vi "ROV_IO 2 (SubVI).vi"(11 "ROV string":string="34.5,,,,$56.3,34.556,,,,$67.9") -> (3 "ROV OK":string)   [LabVIEW 2014]
panel:
  out "ROV temp":string
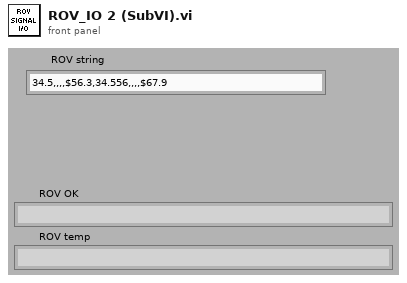
[diagram p1: front panel]
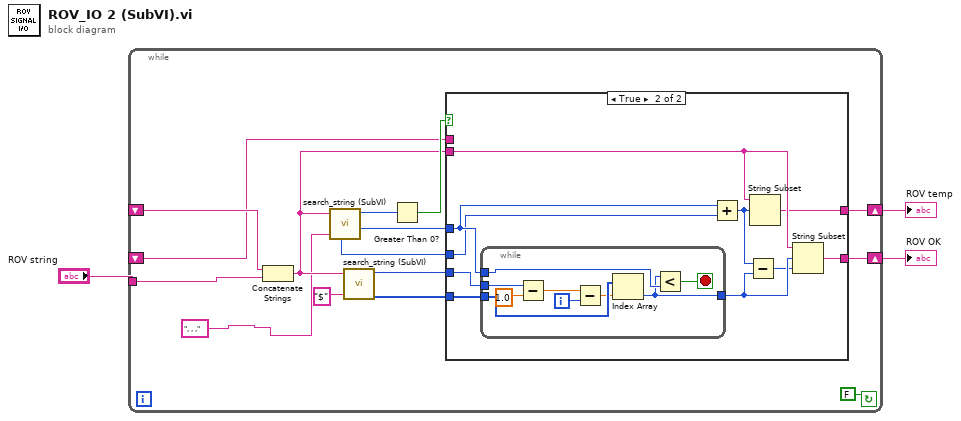
[diagram p0: block diagram]
diagram:
  n1 = while {
    tunnel: "ROV string" -> [w5]
    shift-right: [w9] -> w2
    shift-left: _ -> [w6]
    shift-right: [w8] -> w1
    shift-left: _ -> [w7]
    stop <- FALSE continue-if-true
    n2 = Concatenate Strings(w7, w5) -> (w11:string)
    n3 = call "search_string (SubVI).vi"("string"=w11, "search string/char (-)"=", , ,") -> ("search length"=w10:i32, "no. hits"=w16:i32, "pos last"=w12:i32)  [unwired: 6 out]
    n4 = call "search_string (SubVI).vi"("string"=w11, "search string/char (-)"="$") -> ("no. hits"=w14:i32, "pos vec"=w13:i32[])  [unwired: 7 out]
    n5 = Greater Than 0?(x=w16) -> (x > 0?=w15:bool)
    n6 = case shown="True" w15 {
      tunnel: w14 -> [_ w29]
      tunnel: w13 -> [_ w30]
      tunnel: w12 -> [_ w28]
      tunnel: w11 -> [w19 w23]
      tunnel: w10 -> [_ w27]
      tunnel: [w20 w24] -> w9
      tunnel: [w19 w22] -> w8
      tunnel: w6 -> [w20 _]
      frame False {
      }
      frame True {
        n7 = while {
          tunnel: w30 -> [w39]
          tunnel: w29 -> [w37]
          tunnel: w28 -> [w33]
          tunnel: [w31] -> w26
          i -> [w36]
          stop <- w32 stop-if-true
          n8 = Subtract(x=w37, y=1.0) -> (x-y=w35:dbl)
          n9 = Subtract(x=w35, y=w36) -> (x-y=w34:dbl)
          n10 = Index Array(array=w39, index=w34) -> (element=w31:i32)
          n11 = Less?(x=w31, y=w33) -> (x < y?=w32:bool)
        }
        n12 = Add(x=w28, y=w27) -> (x+y=w21:i32)
        n13 = Subtract(x=w21, y=w26) -> (x-y=w25:i32)
        n14 = String Subset(string=w23, offset (0)=w21) -> (substring=w22:string)  [unwired: 1 in]
        n15 = String Subset(string=w23, offset (0)=w26, length (rest)=w25) -> (substring=w24:string)
      }
    }
  }
  "ROV OK" <- w2
  "ROV temp" <- w1
